vi "Weather Station UI.vi"(7 "stop":bool, 9 "Lower Limit":dbl=10.0 min=0.0 max=50.0, 10 "Upper Limit":dbl=30.0 min=0.0 max=50.0) -> (1 "Warning":string, 2 "Temperature History":dbl(graph))   [LabVIEW 2014]
doc: "This is the main VI in the Weather Station Project. It contains the user interface for a temperature warning system. Temperature is retrieved every half second; data is logged when a warning has occurred.\n\nUser inputs: Temperature Upper Limit, Temperature Lower Limit, Temperature Units.\nOutputs: Current Temperature, Warning State"
uses:
  Supporting Files/Weather Station States.ctl
  Instance           2 26Saved   Weather Station UI .vi
panel:
  # "Temperature Ranges (C)"
  # "Heat \nStroke"
  # "Freeze"
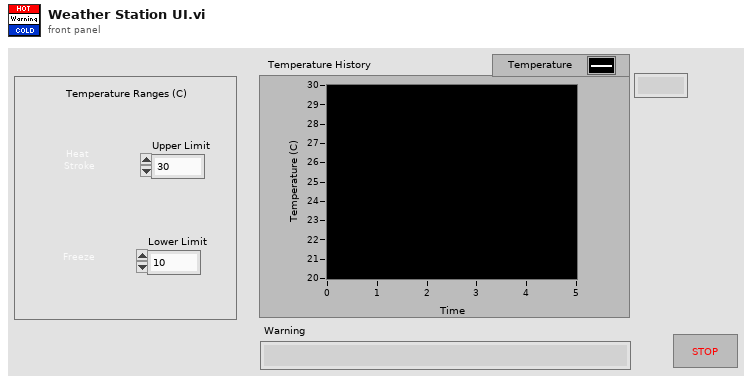
[diagram p1: front panel]
types:
  T1 = enum16{"open", "replace", "create", "open or create", "replace or create", "replace or create with confirmation"}
  T2 = typedef "Weather Station States.ctl" = enum16{"Acquisition", "Range Check", "Analysis", "Data Log", "Time Check"}
  T3 = cluster{"Temperature":dbl, "T Upper Limit":dbl, "T Lower Limit":dbl, "Warning":string}
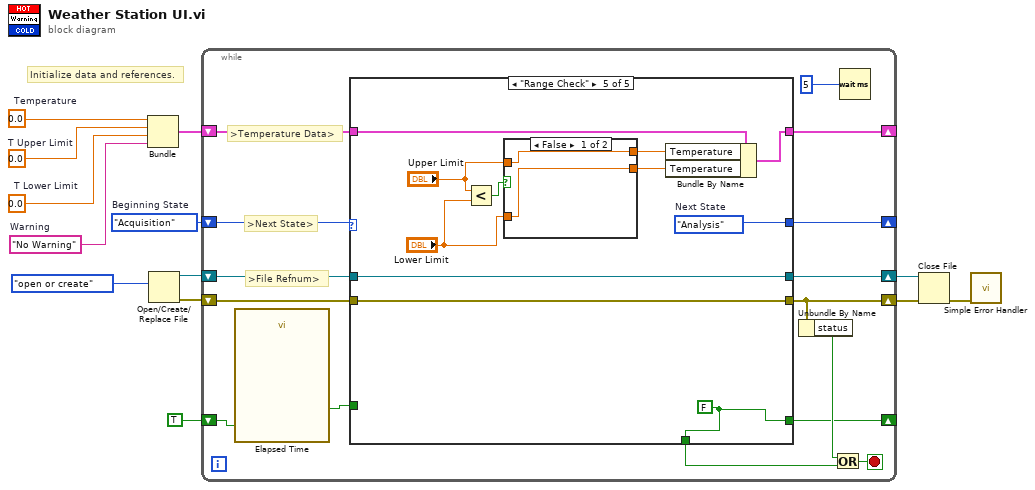
[diagram p0: block diagram]
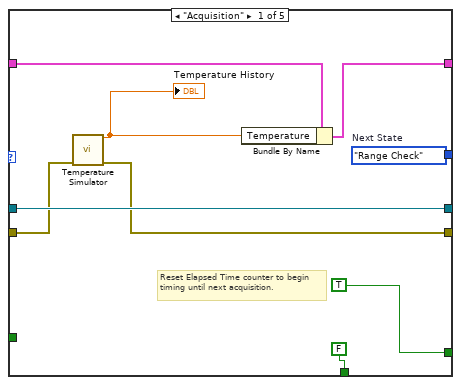
[diagram p2: hidden frame]
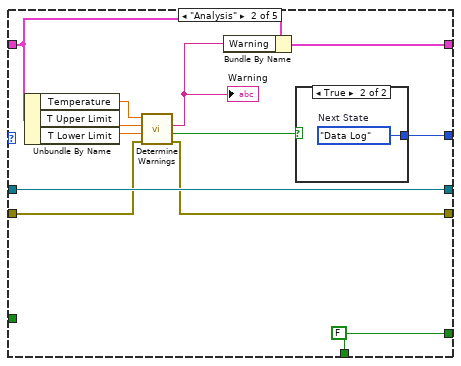
[diagram p3: hidden frame]
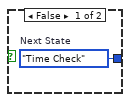
[diagram p4: hidden frame]
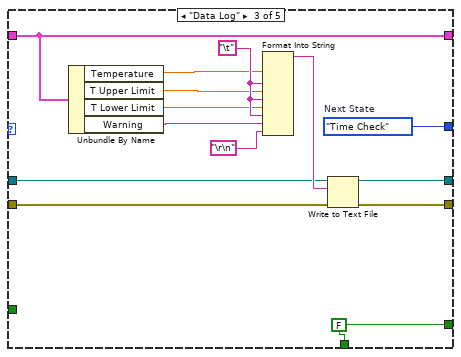
[diagram p5: hidden frame]
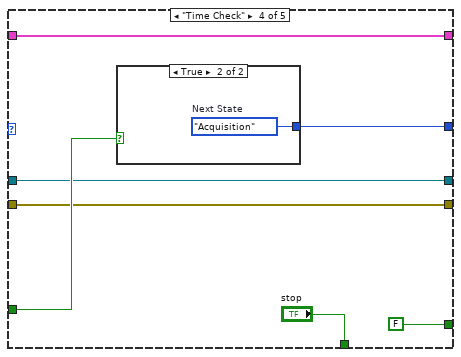
[diagram p6: hidden frame]
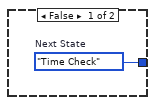
[diagram p7: hidden frame]
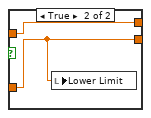
[diagram p8: hidden frame]
diagram:
  w7 = 0.0  # T Lower Limit
  w6 = 0.0  # T Upper Limit
  w8 = "No Warning"  # Warning
  w4 = 0.0  # Temperature
  w13 = Weather_Station_States."Acquisition"  # Beginning State
  # "Initialize data and references."
  n1 = Bundle("Temperature"=w4, "T Upper Limit"=w6, "T Lower Limit"=w7, "Warning"=w8) -> (w1:T3)  [unwired: 1 in]
  n2 = Open/Create/Replace File(operation (0:open)=T1."open or create") -> (refnum out=w3:refnum<file>, error out=w2:errorcluster)  [unwired: 5 in, 1 out]
  n3 = while {
    shift-right: [w27] -> _
    shift-left: w13 -> [w28]
    shift-right: [w14] -> w12
    shift-left: w2 -> [w26]
    shift-right: [w15] -> _
    shift-left: w1 -> [w22]
    shift-right: [w23] -> w11
    shift-left: w3 -> [w21]
    shift-right: [w16] -> _
    shift-left: TRUE ("stop") -> [w18]
    stop <- w25 stop-if-true
    # ">Temperature Data>"
    # ">File Refnum>"
    # ">Next State>"
    n4 = call "Elapsed Time"("Reset"=w18) -> ("Time has Elapsed"=w17:bool)  [unwired: 11 in, 7 out]
    n5 = case shown="\"Range Check\"" w28 {
      tunnel: [w37 w47 w65 w71 w82] -> w27
      tunnel: [w31 w40 w63 w67 w85] -> w14
      tunnel: w26 -> [w30 w41 w64 w67 w85]
      tunnel: [w36 w49 w62 w68 w84] -> w23
      tunnel: [w32 w42 w52 w66 w75] -> w15
      tunnel: w22 -> [w33 w43 w52 w66 w76]
      tunnel: w21 -> [w36 w49 w60 w68 w84]
      tunnel: [FALSE ("stop") w48 w58 "stop" w83] -> w20
      tunnel: w17 -> [_ _ _ w72 _]
      tunnel: [TRUE ("stop") w48 w58 FALSE ("stop") w83] -> w16
      frame "Acquisition" {
        w37 = Weather_Station_States."Range Check"  # Next State
        # "Reset Elapsed Time counter to begin timing until next acquisition."
        n6 = call "Temperature Simulator.vi"("error in (no error)"=w30) -> ("data"=w29:dbl, "error out"=w31:errorcluster)  [unwired: 13 in]
        "Temperature History" <- w29
        n7 = Bundle By Name(cluster=w33, "Temperature"=w29) -> (w32:T3)
      }
      frame "Analysis" {
        w48 = FALSE ("stop")
        n8 = Unbundle By Name(w43) -> ("Temperature"=w46:dbl, "T Upper Limit"=w45:dbl, "T Lower Limit"=w44:dbl)
        n9 = call "Determine Warnings.vi"("error in (no error)"=w41, "Min Temp"=w44, "Max Temp"=w45, "Current Temp"=w46) -> ("error out"=w40:errorcluster, "Warning?"=w38:bool, "Warning Text"=w39:string)  [unwired: 5 in]
        "Warning" <- w39
        n10 = Bundle By Name(cluster=w43, "Warning"=w39) -> (w42:T3)
        n11 = case shown="True" w38 {
          tunnel: [w50 w51] -> w47
          frame False {
            w50 = Weather_Station_States."Time Check"  # Next State
          }
          frame True {
            w51 = Weather_Station_States."Data Log"  # Next State
          }
        }
      }
      frame "Data Log" {
        w65 = Weather_Station_States."Time Check"  # Next State
        w58 = FALSE ("stop")
        w59 = "\t"
        n12 = Unbundle By Name(w52) -> ("Temperature"=w57:dbl, "T Upper Limit"=w56:dbl, "T Lower Limit"=w55:dbl, "Warning"=w54:string)
        n13 = Format Into String(w57, w59, w56, w59, w55, w59, w54, "\r\n") -> (resulting string=w61:string)  [unwired: 3 in, 1 out]
        n14 = Write to Text File(file (use dialog)=w60, text=w61, error in=w64) -> (refnum out=w62:refnum<file>, error out=w63:errorcluster)  [unwired: 1 in, 1 out]
      }
      frame "Time Check" {
        n15 = case shown="True" w72 {
          tunnel: [w73 w74] -> w71
          frame False {
            w73 = Weather_Station_States."Time Check"  # Next State
          }
          frame True {
            w74 = Weather_Station_States."Acquisition"  # Next State
          }
        }
      }
      frame "Range Check" {
        w82 = Weather_Station_States."Analysis"  # Next State
        w83 = FALSE
        n16 = Less?(x="Upper Limit", y="Lower Limit") -> (x < y?=w79:bool)
        n17 = case shown="False" w79 {
          tunnel: "Upper Limit" -> [w87 w89]
          tunnel: "Lower Limit" -> [w86 w88]
          tunnel: [w87 w89] -> w78
          tunnel: [w86 w88] -> w77
          frame False {
          }
          frame True {
            n18 = local write "Lower Limit"(w88) -> ()
          }
        }
        n19 = Bundle By Name(cluster=w76, "Temperature"=w78, "Temperature"=w77) -> (w75:T3)
      }
    }
    n20 = Unbundle By Name(w14) -> ("status"=w24:bool)
    n21 = Or(x=w24, y=w20) -> (x .or. y?=w25:bool)
    n22 = Wait (ms)(milliseconds to wait=u32 5 ("y")) -> ()  [unwired: 1 out]
  }
  n23 = Close File(refnum=w11, error in=w12) -> (error out=w10:errorcluster)  [unwired: 1 out]
  n24 = call <vilib>:"Simple Error Handler.vi"("error in (no error)"=w10) -> ()  [unwired: 4 in, 5 out]
